vi "MI measurements.vi"() -> ()   [LabVIEW 2015]
uses:
  <vilib>/express/express arith-compare/Formula/XNode/ExpressFormulaBlockNode.xnode
  <instrlib>/Rohde&Schwarz Vector Network Analyzer/Rohde&Schwarz Vector Network Analyzer.lvlib
panel:
  in  "1 Hz < IFBW < 1MHz (10 kHz default)":dbl=10000.0 min=1.0 max=10000000.0
  in  "-20 dB < Power < 20 dB (0 dB default)":dbl min=-20.0 max=20.0
  in  "Delay time along ther sample (ps)":dbl min=0.0 max=1000.0
  out "Number of DMM's attempts":i32=1
  out "DMM reading":dbl=5.649249
  out "Current field point":i32=98
  in  "DMM's connection":refnum<visa-resource-name>="Multimeter"
  in  "Choose the folder where the field dependencies of S-parameters and Z will be saved":path=path "C:/Users/ZJUcomposite/Desktop/Tests"
  in  "HMF's connection":refnum<visa-resource-name>="Generator"
  in  "VNA's connection":refnum<visa-resource-name>="ZNB-VNA"
  in  "Coil resistance > 0 (Ohm)":dbl=8.38 min=0.1 max=1000.0
  in  "Coil inductance > 0 (H)":dbl=0.32 min=0.0 max=100.0
  in  "Number of field points (N > 3) for the forward/return sweep":i32=100 min=3 max=1000 step=1
  in  "Volltage to field coefficient > 0 (Oe/V)":dbl=4.29 min=0.0 max=1000.0
  in  "Max input voltage for the amplifier (0<V<2)":dbl=1.5 min=0.0 max=10.0
  in  "Number of frequency points":i32=1 min=1 max=1000
  in  "VNA's port(s) used for measurements":string(combo)="S21"
  # "The procedure measures the field dependencies (including the hysteresis) of S-parameters and Z for the specified frequencies.\n\nVNA must be already calibrated before the measurements. The procedure will not change the calibration but you can modify IFBW and power. \n\nThe frequency values will be entered during the user dialog. All frequency values must be within the frequency range used during the calibration of VNA.\n\nThe voltage to field coefficient (Oe/V) must be found from the coil calibration.\n\nThe maximum number of the field points is 1000 (for each branch of the hysteresis).\n\nThe delay time along the sample must be found separately.\n\nThe coil resistance R and inductance L must be larger than zero. Measure them by a digital multimeter (DMM).\n\nPlease check the maximum input voltage max V allowed for your waveform amplifier. Also the ratio maxV / R must be below the current rate of your waveform amplifier. \n\n******************************************\nDmitriy Makhnovskiy@Hangzhou November 2018\nSensing Materials Technology Ltd, UK\nE-mail: contact@sensmattech.co.uk"
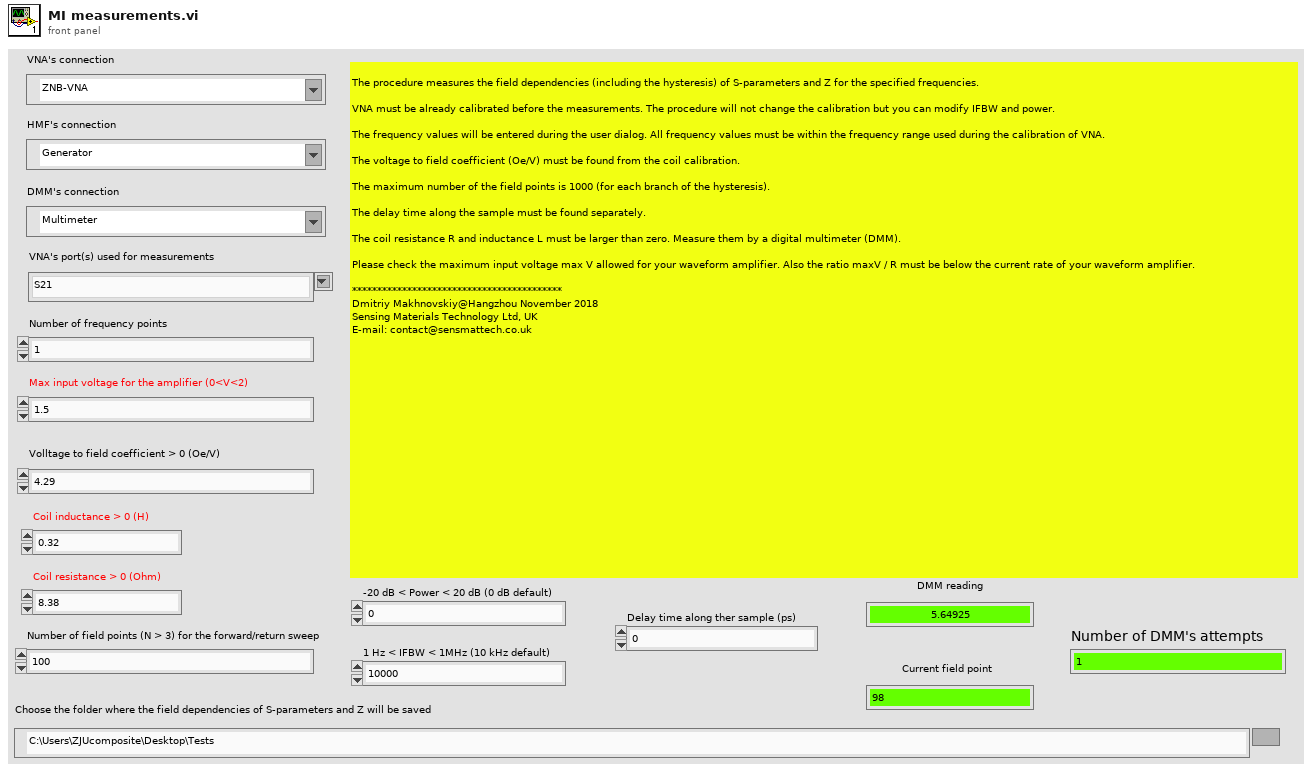
[diagram p1: front panel]
types:
  T1 = typedef "NI_Matrix.lvlib/RealMatrix.ctl" = dbl[][]
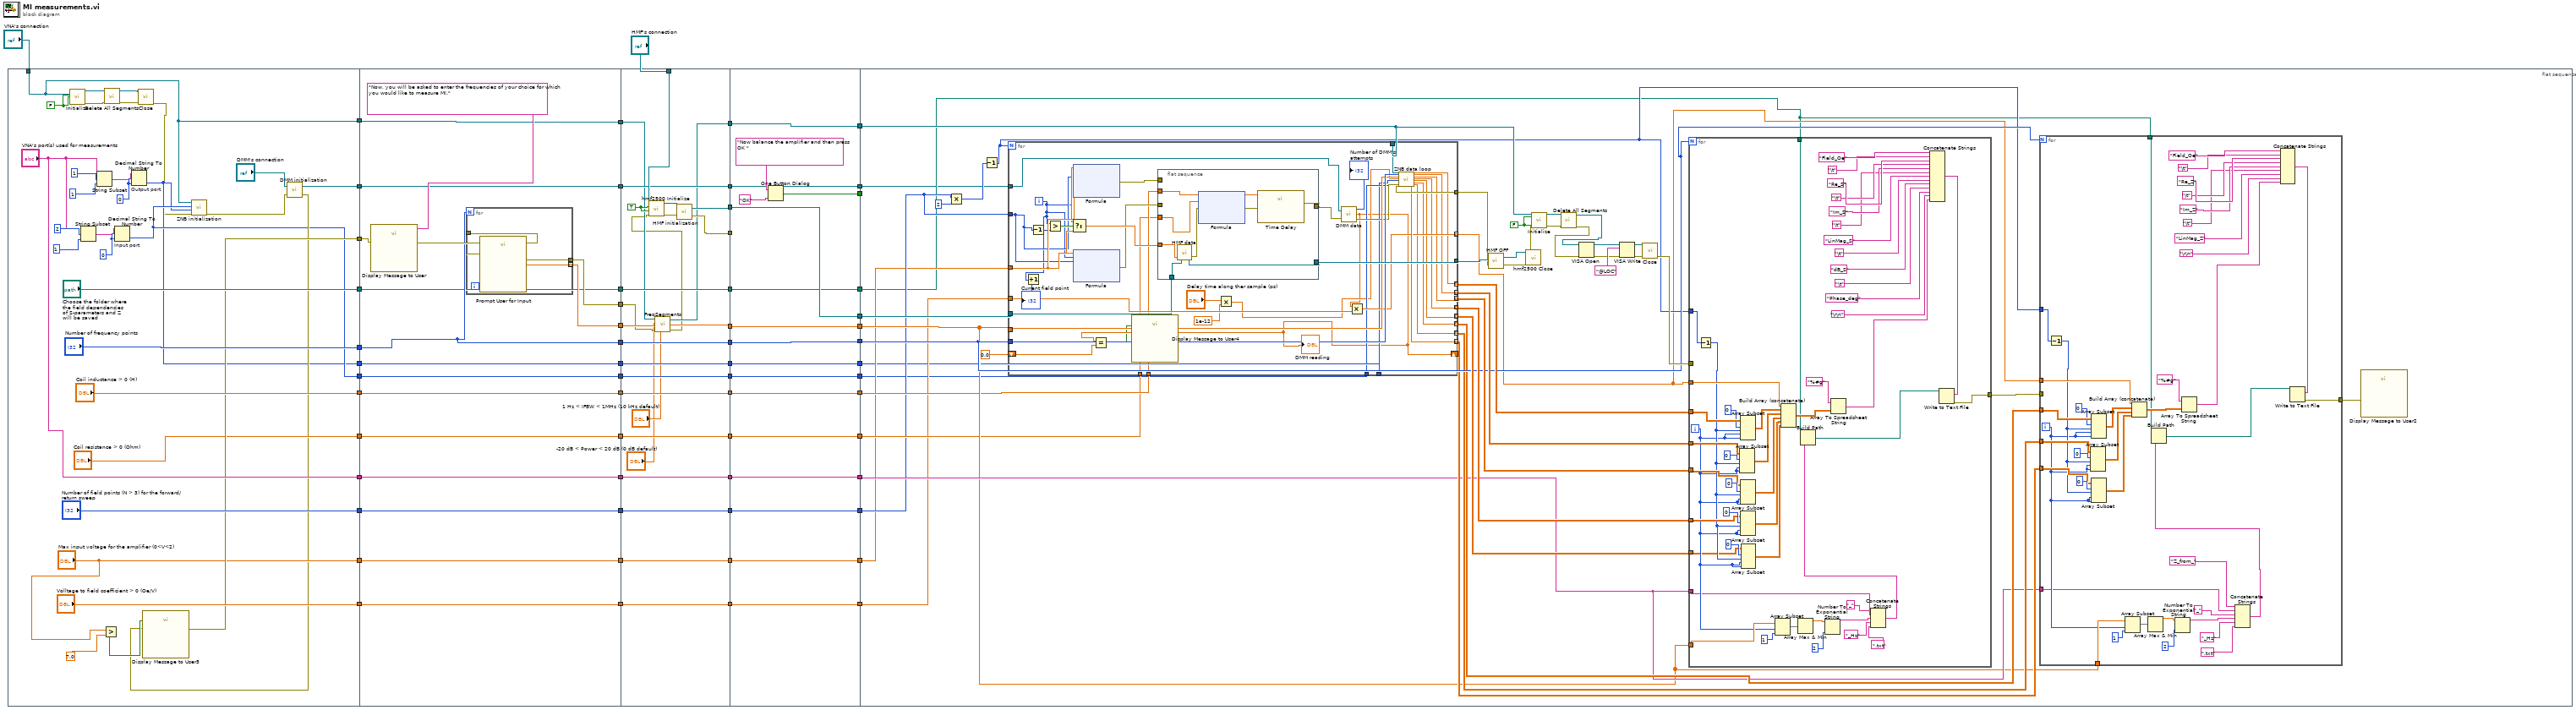
[diagram p0: block diagram]
diagram:
  n1 = flat-sequence {
    tunnel: [w65] -> w46
    tunnel: ["VNA's port(s) used for measurements"] -> w41
    tunnel: "VNA's connection" -> [w65]
    tunnel: ["Number of frequency points"] -> w38
    tunnel: ["Coil inductance > 0 (H)"] -> w34
    tunnel: ["Coil resistance > 0 (Ohm)"] -> w30
    tunnel: ["Number of field points (N > 3) for the forward/return sweep"] -> w26
    tunnel: ["Max input voltage for the amplifier (0<V<2)"] -> w22
    tunnel: ["Volltage to field coefficient > 0 (Oe/V)"] -> w18
    tunnel: ["Choose the folder where the field dependencies of S-parameters and Z will be saved"] -> w14
    tunnel: [w76] -> w13
    tunnel: [w70] -> w9
    tunnel: [w68] -> w5
    tunnel: [w67] -> w1
    tunnel: [w106] -> w56
    tunnel: [w102] -> w54
    tunnel: [w105] -> w52
    tunnel: [w104] -> w47
    tunnel: w46 -> [w104]
    tunnel: [w103] -> w42
    tunnel: w41 -> [w103]
    tunnel: w38 -> [w102]
    tunnel: [w101] -> w35
    tunnel: w34 -> [w101]
    tunnel: [w100] -> w31
    tunnel: w30 -> [w100]
    tunnel: [w99] -> w27
    tunnel: w26 -> [w99]
    tunnel: [w98] -> w23
    tunnel: w22 -> [w98]
    tunnel: [w97] -> w19
    tunnel: w18 -> [w97]
    tunnel: [w96] -> w15
    tunnel: w14 -> [w96]
    tunnel: w13 -> [w95]
    tunnel: [w94] -> w10
    tunnel: w9 -> [w94]
    tunnel: [w93] -> w6
    tunnel: w5 -> [w93]
    tunnel: [w92] -> w2
    tunnel: w1 -> [w92]
    tunnel: w56 -> [w119]
    tunnel: [w118] -> w55
    tunnel: w54 -> [w136]
    tunnel: [w136] -> w53
    tunnel: w52 -> [w114]
    tunnel: [w132] -> w51
    tunnel: [w116] -> w48
    tunnel: w47 -> [w117]
    tunnel: [w120] -> w45
    tunnel: [w131] -> w43
    tunnel: w42 -> [w131]
    tunnel: "HMF's connection" -> [w130]
    tunnel: [w129] -> w36
    tunnel: w35 -> [w129]
    tunnel: [w128] -> w32
    tunnel: w31 -> [w128]
    tunnel: [w127] -> w28
    tunnel: w27 -> [w127]
    tunnel: [w126] -> w24
    tunnel: w23 -> [w126]
    tunnel: [w125] -> w20
    tunnel: w19 -> [w125]
    tunnel: [w124] -> w16
    tunnel: w15 -> [w124]
    tunnel: [w123] -> w11
    tunnel: w10 -> [w123]
    tunnel: [w122] -> w7
    tunnel: w6 -> [w122]
    tunnel: [w121] -> w3
    tunnel: w2 -> [w121]
    tunnel: [w151] -> w59
    tunnel: w55 -> [w150]
    tunnel: [w150] -> w58
    tunnel: w53 -> [w149]
    tunnel: [w149] -> w57
    tunnel: w51 -> [w148]
    tunnel: [w148] -> w50
    tunnel: [w147] -> w49
    tunnel: w48 -> [w147]
    tunnel: w45 -> [_]
    tunnel: [w146] -> w44
    tunnel: w43 -> [w146]
    tunnel: [w145] -> w37
    tunnel: w36 -> [w145]
    tunnel: [w144] -> w33
    tunnel: w32 -> [w144]
    tunnel: [w143] -> w29
    tunnel: w28 -> [w143]
    tunnel: [w142] -> w25
    tunnel: w24 -> [w142]
    tunnel: [w141] -> w21
    tunnel: w20 -> [w141]
    tunnel: [w140] -> w17
    tunnel: w16 -> [w140]
    tunnel: [w139] -> w12
    tunnel: w11 -> [w139]
    tunnel: [w138] -> w8
    tunnel: w7 -> [w138]
    tunnel: [w137] -> w4
    tunnel: w3 -> [w137]
    tunnel: w59 -> [_]
    tunnel: w58 -> [w170]
    tunnel: w57 -> [w178]
    tunnel: w50 -> [w197]
    tunnel: w49 -> [w187]
    tunnel: w44 -> [w171]
    tunnel: w37 -> [w168]
    tunnel: w33 -> [w167]
    tunnel: w29 -> [w166]
    tunnel: w25 -> [w165]
    tunnel: w21 -> [w164]
    tunnel: w17 -> [w163]
    tunnel: w12 -> [w162]
    tunnel: w8 -> [w160]
    tunnel: w4 -> [w159]
    frame #0 {
      w83 = FALSE
      w91 = 0
      w87 = 0
      n2 = call <instrlib>:"Initialize.vi"("VISA resource name"=w65, "ID Query (T: Check)"=w83, "Reset (T: Reset)"=w83) -> ("VISA resource name out"=w61:refnum<visa-resource-name>, "error out"=w63:errorcluster)  [unwired: 11 in]
      n3 = String Subset(string="VNA's port(s) used for measurements", offset (0)=2, length (rest)=1) -> (substring=w90:string)
      n4 = String Subset(string="VNA's port(s) used for measurements", offset (0)=1, length (rest)=1) -> (substring=w86:string)
      n5 = Greater?(x="Max input voltage for the amplifier (0<V<2)", y=7.0) -> (0:w73:bool)
      n6 = call <instrlib>:"Delete All Segments.vi"("error in (no error)"=w63, "VISA resource name"=w61) -> ("error out"=w62:errorcluster, "VISA resource name out"=w60:refnum<visa-resource-name>)  [unwired: 8 in]
      n7 = Decimal String To Number "Input port"(string=w90, offset=w91, default (0L)=w91) -> (number=w68:i32)  [unwired: 1 out]
      n8 = Decimal String To Number "Output port"(string=w86, offset=w87, default (0L)=w87) -> (number=w67:i32)  [unwired: 1 out]
      n9 = call <instrlib>:"Close.vi"("error in (no error)"=w62, "VISA resource name"=w60) -> ("error out"=w64:errorcluster)  [unwired: 9 in]
      n10 = call "ZNB initialization.vi"("error in (no error)"=w64, "Output port"=w67, "Input port"=w68, "VISA resource name"=w65) -> ("error out"=w66:errorcluster)  [unwired: 7 in]
      n11 = call "DMM initialization.vi"("error in (no error)"=w66, "VISA resource name"="DMM's connection") -> ("error out"=w69:errorcluster, "VISA resource name out"=w70:refnum<visa-resource-name>)
      n12 = call "Display Message to User3"("error in (no error)"=w69, "Enable"=w73) -> ("error out"=w76:errorcluster)  [unwired: 8 in, 1 out]
    }
    frame #1 {
      n13 = call "Display Message to User"("error in (no error)"=w95, "Message"="Now, you will be asked to enter the frequencies of your choice for which you would like to measure MI.") -> ("error out"=w107:errorcluster)  [unwired: 8 in, 1 out]
      n14 = for {
        N: w102 -> [_]
        tunnel: [w111] -> w105
        tunnel: w107 -> [w110]
        tunnel: [w109] -> w106 mode=indexing
        n15 = call "Prompt User for Input"("error in (no error)"=w110) -> ("Frequency"=w109:dbl, "error out"=w111:errorcluster)  [unwired: 16 in, 1 out]
      }
    }
    frame #2 {
      w135 = TRUE
      n16 = call "FreqSegments.vi"("VISA resource name"=w117, "FrequenciesIn"=w119, "Power"="-20 dB < Power < 20 dB (0 dB default)", "error in (no error)"=w114, "IFBW"="1 Hz < IFBW < 1MHz (10 kHz default)") -> ("VISA resource name out"=w116:refnum<visa-resource-name>, "FrequenciesOut"=w118:dbl[], "error out"=w115:errorcluster)
      n17 = call <instrlib>:"hmf2500 Initialize.vi"("error in (no error)"=w115, "Reset (Reset)"=w135, "ID Query (Check)"=w135, "VISA resource name"=w130) -> ("error out"=w133:errorcluster, "VISA resource name out"=w134:refnum<visa-resource-name>)  [unwired: 6 in]
      n18 = call "HMF initialization.vi"("error in (no error)"=w133, "VISA resource name"=w134) -> ("error out"=w120:errorcluster, "VISA resource name out"=w132:refnum<visa-resource-name>)
    }
    frame #3 {
      n19 = One Button Dialog(message="Now balance the amplifier and then press OK ", button name ("OK")="OK") -> (true=w151:bool)
    }
    frame #4 {
      w185 = FALSE
      n20 = Multiply(x=w166, y=2) -> (x*y=w193:i32)
      n21 = Decrement(x=w193) -> (x-1=w177:i32)
      n22 = for {
        N: w177 -> [_]
        tunnel: w165 -> [w327]
        tunnel: w164 -> [w325]
        tunnel: w166 -> [w317]
        tunnel: w178 -> [w315]
        tunnel: [w311] -> w175 mode=indexing
        tunnel: w197 -> [w320]
        tunnel: [w319] -> w196
        tunnel: w187 -> [w316]
        tunnel: w170 -> [w314]
        tunnel: [w312] -> w172 mode=indexing
        tunnel: [w313] -> w161
        tunnel: [w310] -> w173 mode=indexing
        tunnel: [w309] -> w174 mode=indexing
        tunnel: [w308] -> w179 mode=indexing
        tunnel: [w307] -> w180 mode=indexing
        tunnel: [w306] -> w181 mode=indexing
        tunnel: [w305] -> w182 mode=indexing
        tunnel: [w304] -> w183 mode=indexing
        tunnel: w168 -> [w303]
        tunnel: w167 -> [w302]
        tunnel: w162 -> [w299]
        tunnel: w160 -> [w297]
        tunnel: w159 -> [w296]
        shift-right: [w289] -> _
        shift-left: 0.0 -> [w290]
        i -> [w292]
        n23 = Increment(x=w292) -> (x+1=→"Current field point":i32)
        n24 = Decrement(x=w317) -> (x-1=w318:i32)
        n25 = Greater?(x=w292, y=w318) -> (0:w324:bool)
        n26 = xnode "Formula"("X1"=w327, "X2"=w292, "X3"=w317) -> ("Result"=w328:dbl, "error out"=w321:errorcluster)  [unwired: 1 in]
        n27 = xnode "Formula"("X1"=w327, "X2"=w292, "X3"=w317) -> ("Result"=w326:dbl, "error out"=w322:errorcluster)  [unwired: 1 in]
        n28 = Select(t=w326, s=w324, f=w328) -> (s? t:f=w323:dbl)
        n29 = flat-sequence {
          tunnel: [w337] -> w319
          tunnel: w320 -> [w334]
          tunnel: w321 -> [_]
          tunnel: w322 -> [_]
          tunnel: w323 -> [w333]
          tunnel: [w332] -> w301
          tunnel: w303 -> [w331]
          tunnel: w302 -> [w330]
          frame #0 {
            n30 = call "HMF data.vi"("DC offset"=w333, "VISA resource name"=w334) -> ("error out"=w329:errorcluster, "VISA resource name out"=w337:refnum<visa-resource-name>)  [unwired: 1 in]
            n31 = xnode "Formula"("X1"=w331, "X2"=w330, "error in (no error)"=w329) -> ("Result"=w336:dbl, "error out"=w335:errorcluster)
            n32 = call "Time Delay"("error in (no error)"=w335, "Delay Time (s)"=w336) -> ("error out"=w332:errorcluster)  [unwired: 9 in]
          }
        }
        n33 = Multiply(x="Delay time along ther sample (ps)", y=1e-12) -> (x*y=w293:dbl)
        n34 = call "DMM data.vi"("VISA resource name"=w299, "error in (no error)"=w301) -> ("Number of attempts"=→"Number of DMM's attempts":i32, "Voltage"=w289:dbl, "error out"=w300:errorcluster)
        "DMM reading" <- w289
        n35 = Equal?(x=w289, y=w290) -> (x = y?=w288:bool)
        n36 = call "Display Message to User4"("Enable"=w288) -> ()  [unwired: 9 in, 2 out]
        n37 = Multiply(x=w289, y=w325) -> (x*y=w311:dbl)
        n38 = call "ZNB data loop.vi"("VISA resource name"=w316, "Number of frequency points"=w315, "Frequencies"=w314, "Delay Time"=w293, "Output Port"=w296, "Input Port"=w297, "error in (no error)"=w300) -> ("error out"=w313:errorcluster, "ReS"=w304:dbl[], "ImS"=w305:dbl[], "LinMagS"=w306:dbl[], "dBS"=w307:dbl[], "Phase"=w308:dbl[], "ReZ"=w309:dbl[], "ImZ"=w310:dbl[], "LinMagZ"=w312:dbl[])  [unwired: 12 in]
      }
      n39 = call "HMF OFF.vi"("error in (no error)"=w161, "VISA resource name"=w196) -> ("error out"=w194:errorcluster, "VISA resource name out"=w195:refnum<visa-resource-name>)
      n40 = call <instrlib>:"hmf2500 Close.vi"("error in (no error)"=w194, "VISA resource name"=w195) -> ("error out"=w186:errorcluster)  [unwired: 9 in]
      n41 = call <instrlib>:"Initialize.vi"("VISA resource name"=w187, "ID Query (T: Check)"=w185, "Reset (T: Reset)"=w185, "error in (no error)"=w186) -> ("VISA resource name out"=w157:refnum<visa-resource-name>, "error out"=w158:errorcluster)  [unwired: 10 in]
      n42 = call <instrlib>:"Delete All Segments.vi"("error in (no error)"=w158, "VISA resource name"=w157) -> ("error out"=w156:errorcluster, "VISA resource name out"=w155:refnum<visa-resource-name>)  [unwired: 8 in]
      n43 = VISA Open(error in (no error)=w156, VISA resource name=w155) -> (VISA resource name=w189:refnum<visa-resource-name>, error out=w188:errorcluster)  [unwired: 3 in]
      n44 = VISA Write(VISA resource name=w189, write buffer="@LOC", error in (no error)=w188) -> (VISA resource name out=w191:refnum<visa-resource-name>, error out=w190:errorcluster)  [unwired: 1 out]
      n45 = call <instrlib>:"Close.vi"("error in (no error)"=w190, "VISA resource name"=w191) -> ("error out"=w184:errorcluster)  [unwired: 9 in]
      n46 = for {
        N: w178 -> [_]
        tunnel: w184 -> [_]
        tunnel: w170 -> [w285]
        tunnel: w183 -> [w287]
        tunnel: w175 -> [w282]
        tunnel: w177 -> [w274]
        tunnel: w171 -> [w240]
        tunnel: [w266] -> w176
        tunnel: w163 -> [w265]
        tunnel: w182 -> [w262]
        tunnel: w181 -> [w259]
        tunnel: w180 -> [w256]
        tunnel: w179 -> [w251]
        i -> [w252]
        n47 = Decrement(x=w274) -> (x-1=w253:i32)
        n48 = Array Subset(array=w262, index (row)=0, length (row)=w253, index (col)=w252, length (col)=w252) -> (w264:dbl[][])
        n49 = Array Subset(array=w287, index (row)=0, length (row)=w253, index (col)=w252, length (col)=w252) -> (w281:dbl[][])
        n50 = Array Subset(array=w259, index (row)=0, length (row)=w253, index (col)=w252, length (col)=w252) -> (w261:dbl[][])
        n51 = Array Subset(array=w256, index (row)=0, length (row)=w253, index (col)=w252, length (col)=w252) -> (w258:dbl[][])
        n52 = Array Subset(array=w251, index (row)=0, length (row)=w253, index (col)=w252, length (col)=w252) -> (w255:dbl[][])
        n53 = Array Subset(array=w285, index=w252, length=1) -> (w283:dbl[])
        n54 = Build Array (concatenate)(w282, w281, w264, w261, w258, w255) -> (w273:T1)
        n55 = Array Max & Min(array=w283) -> (max value=w280:dbl)  [unwired: 3 out]
        n56 = Number To Exponential String(number=w280, precision (6)=2) -> (E-format string=w278:string)  [unwired: 2 in]
        n57 = Array To Spreadsheet String(array=w273, 3:"%#g") -> (spreadsheet string=w241:string)  [unwired: 1 in]
        n58 = Concatenate Strings(w240, "_", w278, "_Hz", ".txt") -> (w275:string)
        n59 = Build Path(base path=w265, name or relative path=w275) -> (appended path=w271:path)
        n60 = Concatenate Strings("Field_Oe", "\t", "Re_S", "\t", "Im_S", "\t", "LinMag_S", "\t", "dB_S", "\t", "Phase_deg", "\r\n", w241) -> (w270:string)
        n61 = Write to Text File(file (use dialog)=w271, text=w270) -> (error out=w266:errorcluster)  [unwired: 2 in, 2 out]
      }
      n62 = for {
        N: w178 -> [_]
        tunnel: w170 -> [w236]
        tunnel: w174 -> [w238]
        tunnel: w175 -> [w233]
        tunnel: w177 -> [w226]
        tunnel: w171 -> [w203]
        tunnel: [w218] -> w169
        tunnel: w163 -> [w217]
        tunnel: w173 -> [w214]
        tunnel: w172 -> [w211]
        tunnel: w176 -> [_]
        i -> [w209]
        n63 = Decrement(x=w226) -> (x-1=w210:i32)
        n64 = Array Subset(array=w214, index (row)=0, length (row)=w210, index (col)=w209, length (col)=w209) -> (w216:dbl[][])
        n65 = Array Subset(array=w238, index (row)=0, length (row)=w210, index (col)=w209, length (col)=w209) -> (w232:dbl[][])
        n66 = Array Subset(array=w211, index (row)=0, length (row)=w210, index (col)=w209, length (col)=w209) -> (w213:dbl[][])
        n67 = Array Subset(array=w236, index=w209, length=1) -> (w234:dbl[])
        n68 = Build Array (concatenate)(w233, w232, w216, w213) -> (w225:T1)
        n69 = Array Max & Min(array=w234) -> (max value=w231:dbl)  [unwired: 3 out]
        n70 = Number To Exponential String(number=w231, precision (6)=2) -> (E-format string=w229:string)  [unwired: 2 in]
        n71 = Array To Spreadsheet String(array=w225, 3:"%#g") -> (spreadsheet string=w200:string)  [unwired: 1 in]
        n72 = Concatenate Strings("Z_from_", w203, "_", w229, "_Hz", ".txt") -> (w227:string)
        n73 = Build Path(base path=w217, name or relative path=w227) -> (appended path=w223:path)
        n74 = Concatenate Strings("Field_Oe", "\t", "Re_Z", "\t", "Im_Z", "\t", "LinMag_Z", "\r\n", w200) -> (w222:string)
        n75 = Write to Text File(file (use dialog)=w223, text=w222) -> (error out=w218:errorcluster)  [unwired: 2 in, 2 out]
      }
      n76 = call "Display Message to User2"("error in (no error)"=w169) -> ()  [unwired: 9 in, 2 out]
    }
  }
